vi "Reset Position to Zero.vi"(8 "error in (no error)":errorcluster, 11 "ESM303 in":refnum<class "ESM303.lvclass">) -> (0 "error out":errorcluster, 3 "ESM303 out":refnum<class "ESM303.lvclass">)   [LabVIEW 2018, in "ESM303.lvlib" / "ESM303.lvclass"]
uses:
  ESM303.lvclass
  builds/Force Test Stand/Force Test Stand/Force Test Stand.lvlibp/Force Test Stand.lvclass
  C:/Projects/LabVIEW/In-Progress/Jose Rivero-Diaz/builds/Force Test Stand/Force Test Stand/Force Test Stand.lvlibp/Force Test Stand.lvclass
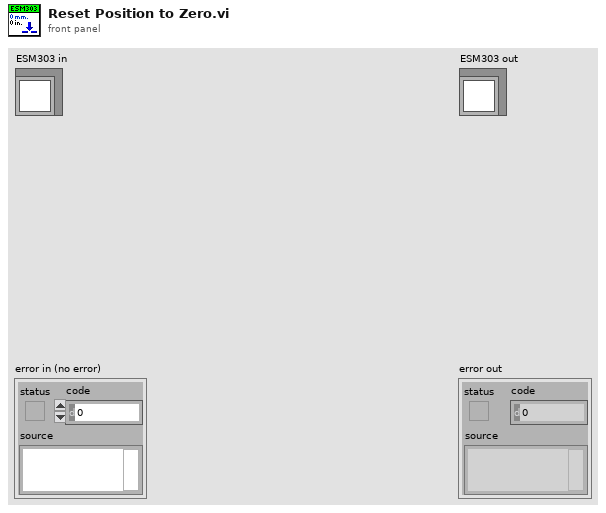
[diagram p1: front panel]
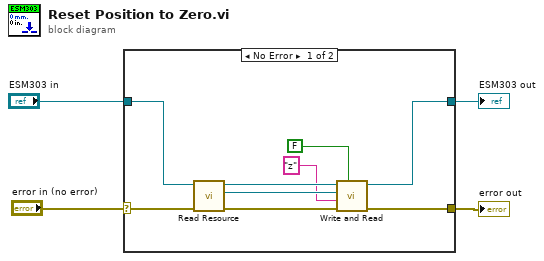
[diagram p0: block diagram]
diagram:
  n1 = case shown="No Error" "error in (no error)" {
    selector: "error in (no error)" -> [w13 w15]
    tunnel: [w5 w15] -> w3
    tunnel: [w6 w14] -> w2
    tunnel: "ESM303 in" -> [w12 w14]
    frame No Error {
      n2 = call "Read Resource.vi"("error in (no error)"=w13, "Force Test Stand in"=w12) -> ("error out"=w11:errorcluster, "Resource"=w9:refnum<visa-resource-name>, "Force Test Stand out"=w10:refnum<class "ESM303.lvclass">)  [unwired: 7 in]
      n3 = call "Write and Read.vi"("Write & Read"=FALSE, "error in (no error)"=w11, "Command"="z", "VISA Refnum in"=w9, "ESM303 in"=w10) -> ("error out"=w5:errorcluster, "ESM303 out"=w6:refnum<class "ESM303.lvclass">)  [unwired: 4 in, 1 out]
    }
    frame Error {
    }
  }
  "error out" <- w3
  "ESM303 out" <- w2
